vi "close.vi"(8 "error in":errorcluster, 11 "TCP":refnum<k5>) -> (0 "error out":errorcluster, 3 "TCP out":refnum<k5>)   [LabVIEW 2025, in "Newtons4thEkg.lvlib"]
uses:
  Newtons4thEkg.lvlib
panel:
  # "Newtons4th V0.10\nClose"
  # "05.05.2025"
  # "Blaz Kelbl"
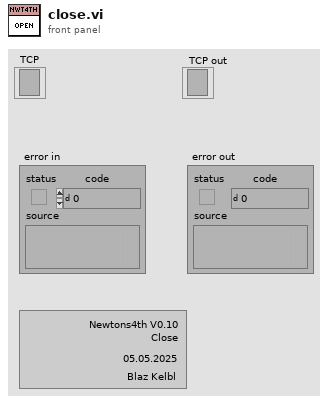
[diagram p1: front panel]
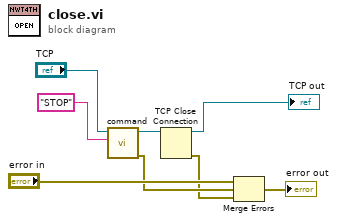
[diagram p0: block diagram]
diagram:
  n1 = call "command.vi"("Query"="STOP", "TCP in"="TCP") -> ("error out"=w2:errorcluster, "TCP out"=w7:refnum<k5>)  [unwired: 7 in, 1 out]
  n2 = TCP Close Connection(connection ID=w7) -> (connection ID out=→"TCP out":refnum<k5>, error out=w1:errorcluster)  [unwired: 2 in]
  n3 = Merge Errors("error in", w2, w1) -> (→"error out":errorcluster)
